vi "RSNRPZ Read Measurement Aux.vi"(8 "error in (no error)":errorcluster, 9 "Timeout (5000 ms)":i32=5000, 10 "Channel (1)":i32=1, 11 "VISA session":refnum<visa-resource-name> caption="VISA resource name") -> (0 "error out":errorcluster, 1 "Aux 1":dbl format="%^.3e", 2 "Measurement":dbl format="%^.3e", 3 "dup VISA session":refnum<visa-resource-name> caption="VISA resource name", 4 "Aux 2":dbl format="%^.3e")   [LabVIEW 2010]
doc: "This VI initiates an acquisition on the channels that you specifies in channel parameter. It then waits for the acquisition to complete, and returns the auxiliary measurement for the channel you specify.\n\nNote(s):\n\n(1) If SENSE:AUX is set to None, this VI returns error."
uses:
  rsnrpz_32.dll
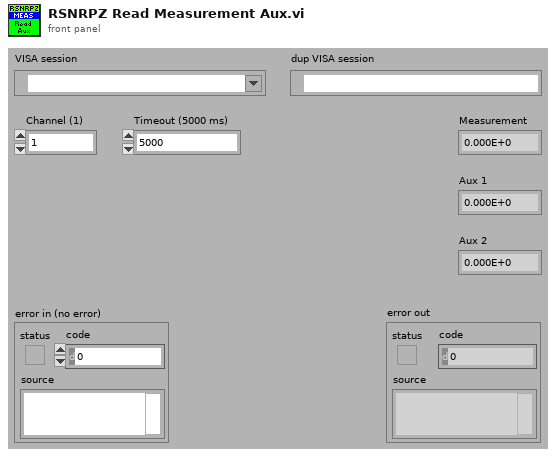
[diagram p1: front panel]
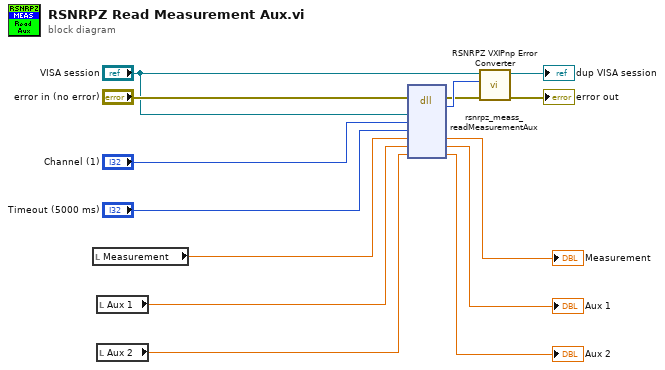
[diagram p0: block diagram]
diagram:
  n1 = local read "Measurement"() -> (w11:dbl)
  n2 = local read "Aux 1"() -> (w9:dbl)
  n3 = local read "Aux 2"() -> (w7:dbl)
  n4 = dll-call lib="rsnrpz_32.dll" fn="rsnrpz_meass_readMeasurementAux"(error in="error in (no error)", "Instrument Handle"="VISA session", "Channel"="Channel (1)", "Timeout (ms)"="Timeout (5000 ms)", "Measurement"=w11, "Aux 1"=w9, "Aux 2"=w7) -> (error out=w5:errorcluster, "Status"=w14:i32, "Measurement"=→"Measurement":dbl, "Aux 1"=→"Aux 1":dbl, "Aux 2"=→"Aux 2":dbl)  [unwired: 5 in, 1 out]
  n5 = call <instrlib>:"RSNRPZ VXIPnp Error Converter.vi"("error in"=w5, "VXIPnp error code"=w14, "VISA session"="VISA session") -> ("error out"=→"error out":errorcluster, "dup VISA session"=→"dup VISA session":refnum<visa-resource-name>)  [unwired: 7 in]
